vi "Get angle range.vi"(8 "error in (no error)":errorcluster, 11 "String":string) -> (0 "error out":errorcluster, 2 "Min":dbl, 3 "Max":dbl)   [LabVIEW 2020]
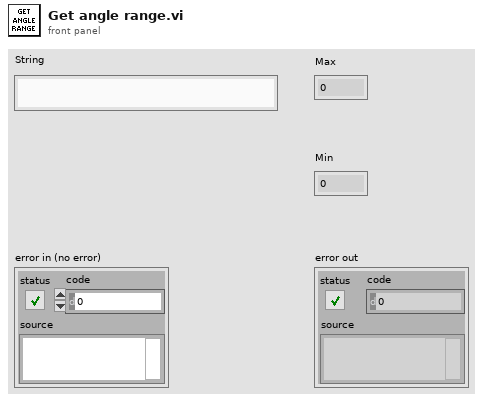
[diagram p1: front panel]
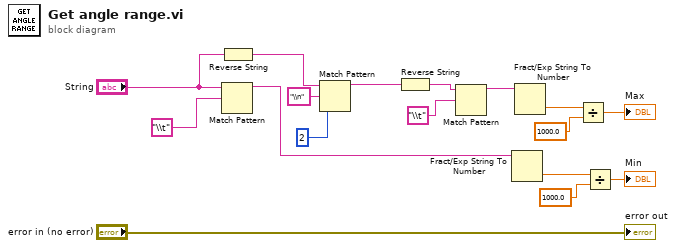
[diagram p0: block diagram]
diagram:
  n1 = Match Pattern(string="String", regular expression="\\t") -> (before substring=w8:string)  [unwired: 1 in, 3 out]
  n2 = Reverse String(1:"String") -> (0:w15:string)
  n3 = Match Pattern(string=w15, regular expression="\\n", offset (0)=2) -> (before substring=w12:string)  [unwired: 3 out]
  n4 = Reverse String(1:w12) -> (0:w11:string)
  n5 = Match Pattern(string=w11, regular expression="\\t" ("string")) -> (before substring=w9:string)  [unwired: 1 in, 3 out]
  n6 = Fract/Exp String To Number(string=w8) -> (number=w3:dbl)  [unwired: 3 in, 1 out]
  n7 = Fract/Exp String To Number(string=w9) -> (number=w7:dbl)  [unwired: 3 in, 1 out]
  n8 = Divide(x=w7, y=1000.0) -> (x/y=→"Max":dbl)
  n9 = Divide(x=w3, y=1000.0) -> (x/y=→"Min":dbl)
  "error out" <- "error in (no error)"
